vi "Init and Verificate Port.vi"(11 "Data Cluster IN":T1={"VISA resource name"="ASRL4::INSTR"}) -> (3 "Data Cluster OUT":T1={"VISA resource name"="ASRL4::INSTR"})   [LabVIEW 2020, in "Serial Device.lvclass"]
uses:
  Serial Device.lvclass
  Data Cluster.ctl
  <vilib>/Instr/_visa.llb/VISA Configure Serial Port (Instr).vi
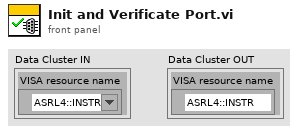
[diagram p1: front panel]
types:
  T1 = typedef "Data Cluster.ctl" = cluster{"VISA resource name":refnum<visa-resource-name>}
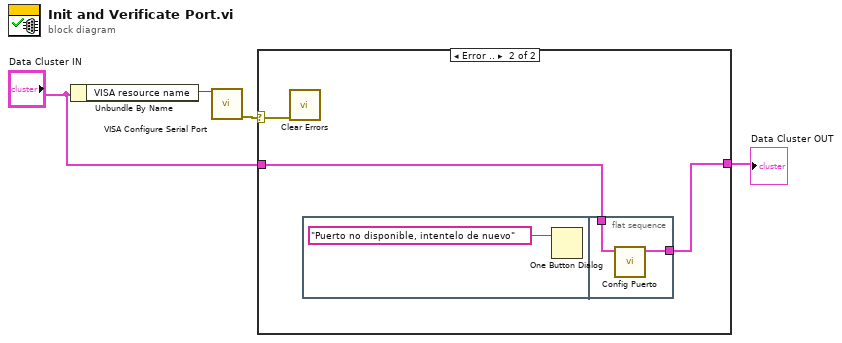
[diagram p0: block diagram]
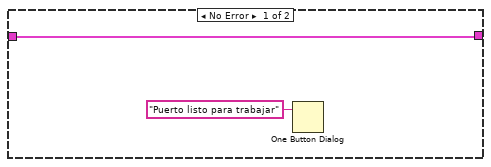
[diagram p2: hidden frame]
diagram:
  n1 = Unbundle By Name("Data Cluster IN") -> ("VISA resource name"=w4:refnum<visa-resource-name>)
  n2 = call-poly "VISA Configure Serial Port"("VISA resource name"=w4) -> ("error out"=w3:errorcluster)  [unwired: 13 in, 1 out]
  n3 = case shown="Error .." w3 {
    selector: w3 -> [_ w9]
    tunnel: "Data Cluster IN" -> [w5 w7]
    tunnel: [w5 w8] -> w1
    frame No Error {
      n4 = One Button Dialog(message="Puerto listo para trabajar") -> ()  [unwired: 1 in, 1 out]
    }
    frame Error {
      n5 = call <vilib>:"Clear Errors.vi"("error in (no error)"=w9) -> ()  [unwired: 5 in, 2 out]
      n6 = flat-sequence {
        tunnel: [w12] -> w8
        tunnel: w7 -> [w11]
        frame #0 {
          n7 = One Button Dialog(message="Puerto no disponible, intentelo de nuevo") -> ()  [unwired: 1 in, 1 out]
        }
        frame #1 {
          n8 = call "Config Puerto.vi"("Data Cluster"=w11) -> ("Data Cluster Out"=w12:T1)  [unwired: 10 in]
        }
      }
    }
  }
  "Data Cluster OUT" <- w1
